vi "PCO_GetCameraHealthStatus.vi"(0 "ph":u64, 11 "error in (no error)":errorcluster {"code" format="%x"}) -> (4 "ph out":u64, 6 "ErrorMessage":i32 format="%x", 8 "dwErr":u32 format="%x", 10 "dwWarn":u32 format="%x", 14 "dwStatus":u32 format="%x", 15 "error out":errorcluster {"code" format="%x"})   [LabVIEW 2019, in "SDK.lvlib" / "GeneralCameraStatus.lvlib"]
doc: "<b>Description:</b>\nThe PCO_GetCameraHealthStatus function retrieves information about the current camera status. The returned parameters are presented as a bit field, where each bit is describing a distinct camera condition. Cleared bits in the bitfield indicate that the particular condition is not valid, set bits show valid (error, warning, status) conditions.\nIn case an error condition is recognized the hardware might get damaged, when operation of the camera is continued. Therefore the application should report the error condition to the user and prompt him to switch off the camera as soon as possible.\nIn case a warning condition is recognized, the operation of the camera can continue, but the image quality might suffer.\nThe status information does give hints about current camera state. It can be determined, if the camera is in the default state (power up), if a PCO_ArmCamera was successfully executed and if camera is currently recording.\nIt is recommended to call this function frequently (e.g. every 5s or after calling PCO_ArmCamera) in order to recognize camera internal problems. This helps to prevent camera hardware from damage.\n\n<b>Supported camera type:</b>\nAll cameras\n\n<b>Descriptor dependency:</b>\nNone"
uses:
  GeneralCameraStatus.lvlib
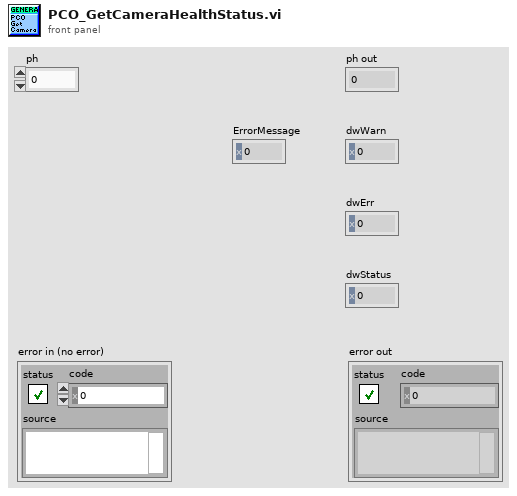
[diagram p1: front panel]
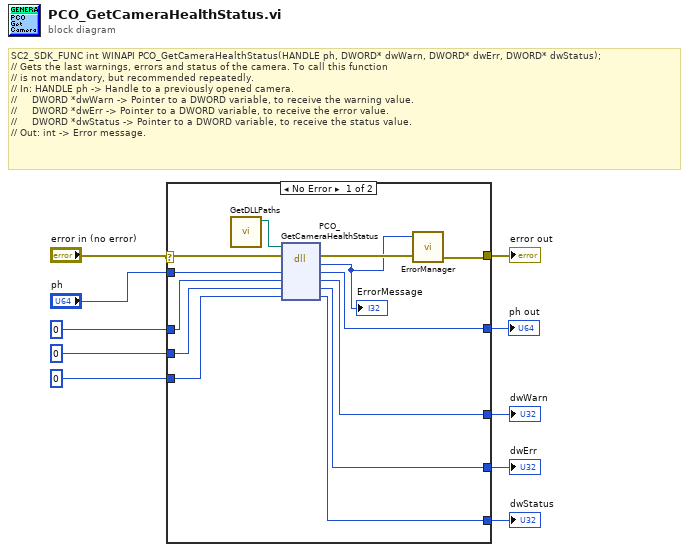
[diagram p0: block diagram]
diagram:
  # "SC2_SDK_FUNC int WINAPI PCO_GetCameraHealthStatus(HANDLE ph, DWORD* dwWarn, DWORD* dwErr, DWORD* dwStatus);\n// Gets the last warnings, errors and status of the camera. To call this function\n// is not mandatory, but recommended repeatedly.\n// In: HANDLE ph -> Handle to a previously opened camera.\n//     DWORD *dwWarn -> Pointer to a DWORD variable, to receive the warning value.\n//     DWORD *dwErr -> Pointer to a DWORD variable, to receive the error value.\n//     DWORD *dwStatus -> Pointer to a DWORD variable, to receive the status value.\n// Out: int -> Error message."
  n1 = case shown="No Error" "error in (no error)" {
    selector: "error in (no error)" -> [w21 w28]
    tunnel: [w22 w28] -> w10
    tunnel: "ph" -> [w20 w27]
    tunnel: [w19 w27] -> w7
    tunnel: [w17 w24] -> w6
    tunnel: [w16 w25] -> w5
    tunnel: [w15 w26] -> w4
    tunnel: u32 0 -> [w14 w26]
    tunnel: u32 0 -> [w13 w25]
    tunnel: u32 0 -> [w12 w24]
    frame No Error {
      n2 = call "GetDLLPaths.vi"() -> ("SC2_Cam_Path"=w11:path)  [unwired: 8 in, 3 out]
      n3 = dll-call lib="?" fn="PCO_GetCameraHealthStatus"(path in=w11, error in=w21, "ph"=w20, "dwWarn"=w14, "dwErr"=w13, "dwStatus"=w12) -> (error out=w23:errorcluster, "return type"=w18:i32, "ph"=w19:u64, "dwWarn"=w15:u32, "dwErr"=w16:u32, "dwStatus"=w17:u32)  [unwired: 1 in, 1 out]
      "ErrorMessage" <- w18
      n4 = call "ErrorManager.vi"("error in (no error)"=w23, "error code"=w18) -> ("error out"=w22:errorcluster)  [unwired: 2 in, 1 out]
    }
    frame Error {
    }
  }
  "error out" <- w10
  "ph out" <- w7
  "dwWarn" <- w4
  "dwErr" <- w5
  "dwStatus" <- w6
